vi "Measurement.vi"() -> ()   [LabVIEW 2014]
uses:
  C:/Users/ThomasNelson/Projects/examples/libraries/bin/visual .net/KClmtrWrapper.dll
  libraries/bin/visual .net/KClmtrWrapper.dll
panel:
  out "Cluster":cluster{"x":dbl, "L":dbl, "y":dbl}
  in  "Port Number":i32=3
  in  "Stop":bool
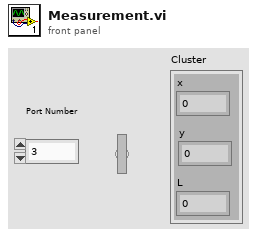
[diagram p1: front panel]
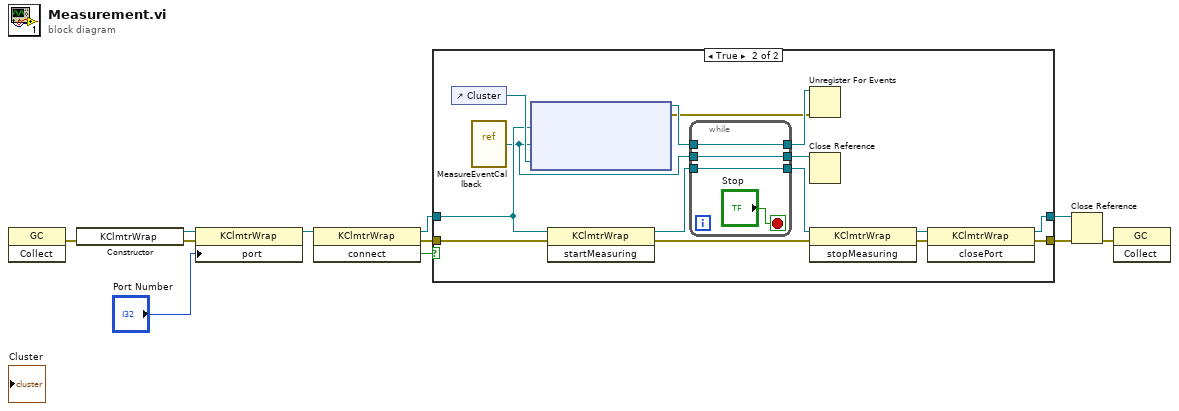
[diagram p0: block diagram]
diagram:
  n1 = invoke class="GC" method="Collect"() -> (error out=w1:errorcluster)  [unwired: 3 in, 2 out]
  n2 = constructor class="KClmtrWrap"(error in=w1) -> (reference out=w11:refnum<k24>, error out=w10:errorcluster)  [unwired: 2 in, 1 out]
  n3 = property class="KClmtrWrap"(reference=w11, error in=w10, "port"="Port Number") -> (reference out=w8:refnum<k24>)  [unwired: 1 out]
  n4 = invoke class="KClmtrWrap" method="connect"(reference=w8) -> (reference out=w5:refnum<k24>, error out=w4:errorcluster, "connect"=w3:bool)  [unwired: 2 in]
  n5 = case shown="True" w3 {
    tunnel: w5 -> [w13 w18]
    tunnel: w4 -> [w12 w17]
    tunnel: [w13 w28] -> w7
    tunnel: [w12 w27] -> w6
    frame False {
    }
    frame True {
      n6 = control-ref of="Cluster"() -> (w21:refnum<vi>)
      n7 = vi-ref "MeasureEventCallback.vi"() -> ("vi reference"=w15:refnum<vi>)
      n8 = node(w18, w15, w21) -> (w22:refnum<k27>, w20:errorcluster)  [unwired: 2 in]
      n9 = invoke class="KClmtrWrap" method="startMeasuring"(reference=w18, error in=w17) -> (reference out=w19:refnum<k24>, error out=w26:errorcluster)  [unwired: 1 in, 1 out]
      n10 = while {
        tunnel: w19 -> [w31]
        tunnel: [w31] -> w25
        tunnel: [w30] -> w23
        tunnel: w22 -> [w30]
        tunnel: w15 -> [w29]
        tunnel: [w29] -> w14
        stop <- "Stop" stop-if-true
      }
      n11 = Unregister For Events(event registration refnum=w23, error in=w20) -> ()  [unwired: 1 out]
      n12 = Close Reference(reference=w14) -> ()  [unwired: 1 in, 1 out]
      n13 = invoke class="KClmtrWrap" method="stopMeasuring"(reference=w25, error in=w26) -> (reference out=w24:refnum<k24>, error out=w16:errorcluster)  [unwired: 1 in, 1 out]
      n14 = invoke class="KClmtrWrap" method="closePort"(reference=w24, error in=w16) -> (reference out=w28:refnum<k24>, error out=w27:errorcluster)  [unwired: 1 in, 1 out]
    }
  }
  n15 = Close Reference(reference=w7, error in (no error)=w6) -> (error out=w2:errorcluster)
  n16 = invoke class="GC" method="Collect"(error in=w2) -> ()  [unwired: 2 in, 3 out]
